vi "MCB2400 AI Scan PrjAttrValidator.vi"(5 "Ctl Refnum":refnum<vi>, 11 "Attributes":T1 {"Programmable Pin Connections" items=["AI Bank uses AI channels 0-7, which use pins P0.12, P0.13, P0.23, P0.24, P0.25, P0.26, P1.30, and P1.31. You cannot use AI Bank and AI0-7 or these pins in the same project."]}) -> (3 "Valid?":bool)   [LabVIEW 2011]
uses:
  <vilib>/Embedded/ARM/MCB2400/MCB2400_AI_Scan_PrjAttr.ctl
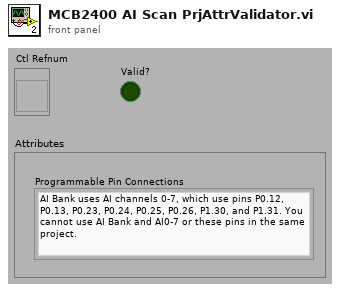
[diagram p1: front panel]
types:
  T1 = typedef "MCB2400_AI_Scan_PrjAttr.ctl" = cluster{"Programmable Pin Connections":u16}
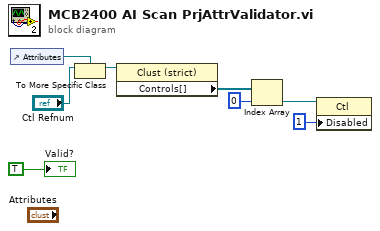
[diagram p0: block diagram]
diagram:
  n1 = control-ref of="Attributes"() -> (w1:refnum<vi>)
  n2 = To More Specific Class(target class=w1, reference="Ctl Refnum") -> (specific class reference=w3:refnum<vi>)  [unwired: 1 in, 1 out]
  n3 = property class="Clust (strict)"(reference=w3) -> ("Controls[]"=w7:refnum<vi>[])  [unwired: 1 in, 2 out]
  n4 = Index Array(array=w7, index=0) -> (element=w5:refnum<vi>)
  n5 = property class="Ctl"(reference=w5, "Disabled"=u8 1) -> ()  [unwired: 1 in, 2 out]
  "Valid?" <- TRUE ("Valid?")
